vi "Crop_ROIs_on_image_boundaries.vi"(8 "error in (no error)":errorcluster, 10 "ROI Descriptor IN":T1 {"Contours"."Type" items=["No Selection", "Point", "Line", "Rectangle", "Oval", "Polygon", "Freehand Region", "Annulus", "Unused2", "Unused3", "Broken Line", "Freehand Line", "Rotated Rectangle"]}, 11 "Image":T2) -> (0 "error out":errorcluster, 2 "ROI Descriptor OUT":T1 {"Contours"."Type" items=["No Selection", "Point", "Line", "Rectangle", "Oval", "Polygon", "Freehand Region", "Annulus", "Unused2", "Unused3", "Broken Line", "Freehand Line", "Rotated Rectangle"]})   [LabVIEW 2012]
uses:
  <vilib>/vision/Image Controls.llb/IMAQ Image.ctl
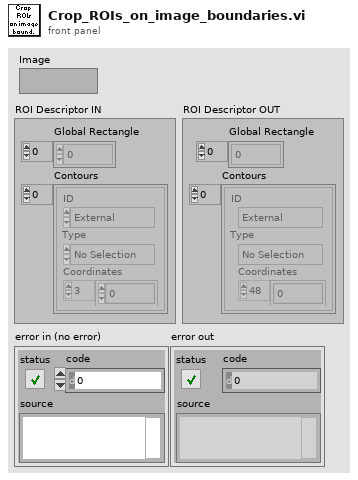
[diagram p1: front panel]
types:
  T1 = typedef "ROI Descriptor" = cluster{"Global Rectangle":i32[], "Contours":cluster{"ID":enum32{"External", "Internal"}, "Type":u32, "Coordinates":i32[]}[]}
  T2 = typedef "IMAQ Image.ctl" = refnum<image>
  T3 = cluster{"ID":enum32{"External", "Internal"}, "Type":u32, "Coordinates":i32[]}[]
  T4 = cluster{"ID":enum32{"External", "Internal"}, "Type":u32, "Coordinates":i32[]}
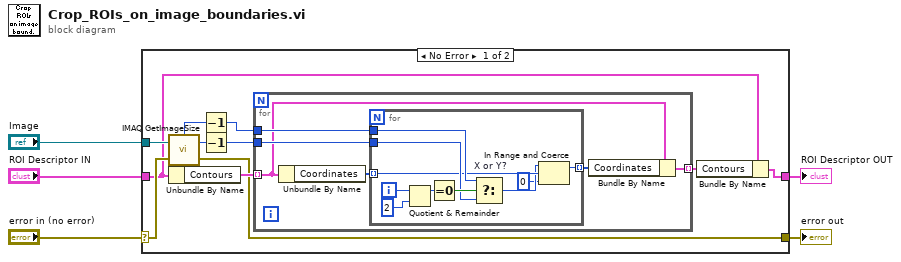
[diagram p0: block diagram]
diagram:
  n1 = case shown="No Error" "error in (no error)" {
    selector: "error in (no error)" -> [w15 w34]
    tunnel: "Image" -> [w16 _]
    tunnel: [w13 w34] -> w3
    tunnel: "ROI Descriptor IN" -> [w12 w33]
    tunnel: [w10 w33] -> w2
    frame No Error {
      n2 = call "IMAQ GetImageSize"("Image"=w16, "error in (no error)"=w15) -> ("Y Resolution"=w8:i32, "X Resolution"=w9:i32, "error out"=w13:errorcluster)  [unwired: 2 in]
      n3 = Unbundle By Name(w12) -> ("Contours"=w14:T3)
      n4 = Decrement(x=w9) -> (x-1=w6:i32)
      n5 = Decrement(x=w8) -> (x-1=w7:i32)
      n6 = for {
        tunnel: w14 -> [w19] mode=indexing
        tunnel: w7 -> [w20]
        tunnel: w6 -> [w21]
        tunnel: [w17] -> w11 mode=indexing
        n7 = Unbundle By Name(w19) -> ("Coordinates"=w22:i32[])
        n8 = for {
          tunnel: w22 -> [w26] mode=indexing
          tunnel: w21 -> [w28]
          tunnel: w20 -> [w27]
          tunnel: [w23] -> w18 mode=indexing
          i -> [w32]
          n9 = Quotient & Remainder(x=w32, y=2) -> (x-y*floor(x/y)=w30:i32)  [unwired: 1 out]
          n10 = Equal To 0?(x=w30) -> (x = 0?=w29:bool)
          n11 = Select "X or Y?"(t=w28, s=w29, f=w27) -> (s? t:f=w25:i32)
          n12 = In Range and Coerce(upper limit=w25, x=w26, lower limit=0) -> (coerced(x)=w23:i32)  [unwired: 1 out]
        }
        n13 = Bundle By Name(cluster=w19, "Coordinates"=w18) -> (w17:T4)
      }
      n14 = Bundle By Name(cluster=w12, "Contours"=w11) -> (w10:T1)
    }
    frame Error {
    }
  }
  "error out" <- w3
  "ROI Descriptor OUT" <- w2
